vi "LEGGI FILE TABELLA.vi"(9 "INDICE TABELLA":u16, 10 "TIPO COLLEGAMENTO":u16) -> (1 "Array INDICI":string[](array[string]), 2 "Array":T1(array[cluster]), 3 "ORDINE":string[][](array[string]))   [LabVIEW 2019]
uses:
  Global percorso impostazioni.vi
  <vilib>/Utility/file.llb/Read Delimited Spreadsheet (string).vi
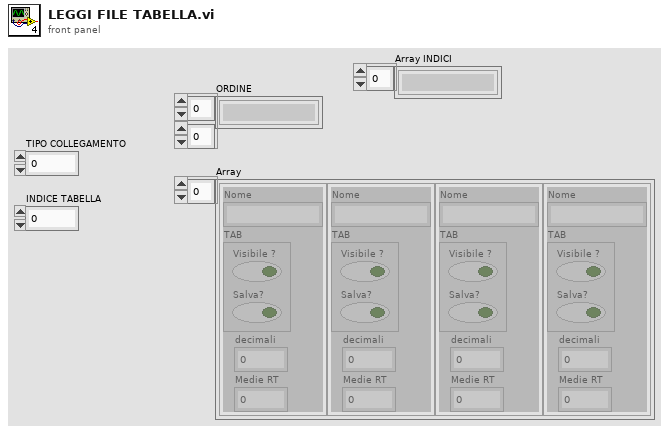
[diagram p1: front panel]
types:
  T1 = cluster{"Nome":string, "TAB":cluster{"Visibile ?":bool, "Salva?":bool}, "decimali":i8, "Medie RT":i8}[]
  T2 = cluster{"Nome":string, "TAB":cluster{"Visibile ?":bool, "Salva?":bool}, "decimali":i8, "Medie RT":i8}
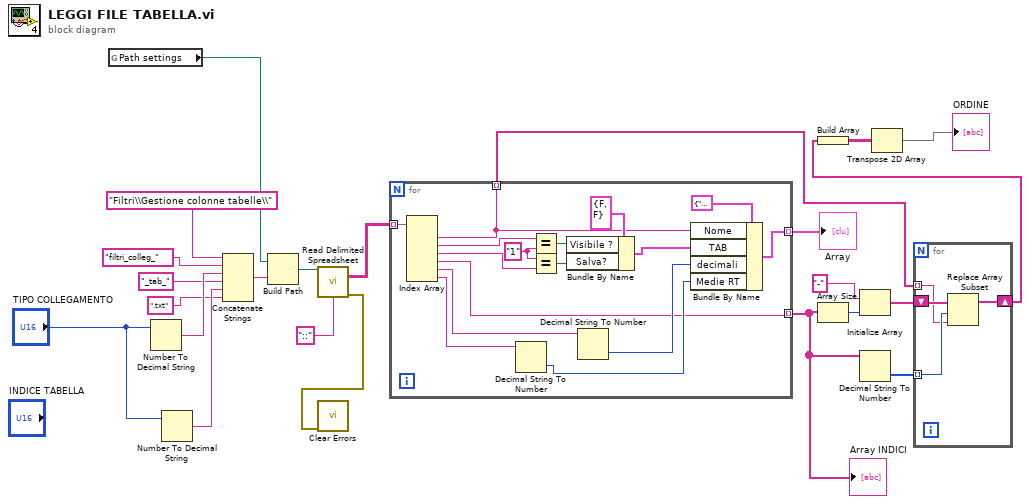
[diagram p0: block diagram]
diagram:
  n1 = global read "Global percorso impostazioni.vi" "Path settings"() -> (w2:path)
  n2 = Number To Decimal String(number="TIPO COLLEGAMENTO") -> (decimal integer string=w19:string)  [unwired: 1 in]
  n3 = Number To Decimal String(number="TIPO COLLEGAMENTO") -> (decimal integer string=w20:string)  [unwired: 1 in]
  n4 = Concatenate Strings("Filtri\\Gestione colonne tabelle\\" ("name or relative path"), "filtri_colleg_" ("string"), w19, "_tab_" ("string"), w20, ".txt" ("string")) -> (w21:string)
  n5 = Build Path(base path=w2, name or relative path=w21) -> (appended path=w22:path)
  n6 = call-poly <vilib>:"Read Delimited Spreadsheet.vi"("file path (dialog if empty)"=w22, "delimiter (\\t)"="::" ("delimiter (\\t)")) -> ("all rows"=w4:string[][], "error out"=w23:errorcluster)  [unwired: 8 in, 4 out]
  n7 = call <vilib>:"Clear Errors.vi"("error in (no error)"=w23) -> ()  [unwired: 5 in, 2 out]
  n8 = for {
    tunnel: [w39] -> w14 mode=indexing
    tunnel: w4 -> [w38] mode=indexing
    tunnel: [w30] -> w10 mode=indexing
    tunnel: [w26] -> w7 mode=indexing
    w33 = "1" ("y")
    n9 = Index Array(array=w38) -> (element #1=w30:string, element #2=w36:string, element #3=w34:string, element #4=w26:string, element #5=w25:string, element #6=w24:string)  [unwired: 6 in]
    n10 = Decimal String To Number(string=w24) -> (number=w28:i32)  [unwired: 2 in, 1 out]
    n11 = Equal?(x=w36, y=w33) -> (x = y?=w37:bool)
    n12 = Equal?(x=w33, y=w34) -> (x = y?=w35:bool)
    n13 = Bundle By Name(cluster=cluster{"Visibile ?":bool, "Salva?":bool} {"Visibile ?"=FALSE, "Salva?"=FALSE} ("QH"), "Visibile ?"=w37, "Salva?"=w35) -> (w32:cluster{"Visibile ?":bool, "Salva?":bool})
    n14 = Decimal String To Number(string=w25) -> (number=w29:i32)  [unwired: 2 in, 1 out]
    n15 = Bundle By Name(cluster=T2 {"Nome"="", "TAB"={"Visibile ?"=FALSE, "Salva?"=FALSE}, "decimali"=0, "Medie RT"=0} ("Cluster"), "Nome"=w30, "TAB"=w32, "decimali"=w29, "Medie RT"=w28) -> (w39:T2)
  }
  "Array" <- w14
  "Array INDICI" <- w7
  n16 = Array Size(array=w7) -> (size(s)=w8:i32)
  n17 = Initialize Array("-", w8) -> (w11:string[])
  n18 = Decimal String To Number(string=w7) -> (number=w9:i32[])  [unwired: 2 in, 1 out]
  n19 = for {
    tunnel: w9 -> [w42] mode=indexing
    tunnel: w10 -> [w41] mode=indexing
    shift-right: [w40] -> w12
    shift-left: w11 -> [w43]
    n20 = Replace Array Subset(array=w43, new element=w41, index=w42) -> (w40:string[])
  }
  n21 = Build Array(w12) -> (w5:string[][])
  n22 = Transpose 2D Array(2D array=w5) -> (transposed array=→"ORDINE":string[][])
